vi "试验判定.vi"(7 "Result":refnum<vi>, 10 "判定参数":T1, 11 "XY曲线":cluster{"X":dbl[], "Y":dbl[]}[](array[cluster])) -> (2 "判定项长度":i32, 3 "OK？":bool)   [LabVIEW 2020]
uses:
  Global_Variable/A131258.vi
  <userlib>/_MGI/1D Array/MGI Average/MGI Average (DBL[]).vi
panel:
  out "逆向平均值":dbl
  out "正向平均值":dbl
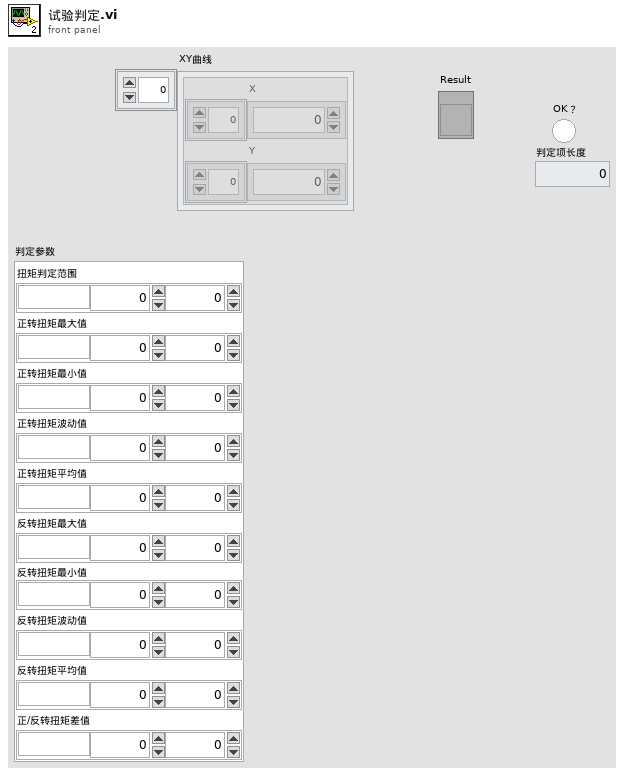
[diagram p1: front panel]
types:
  T1 = cluster{"扭矩判定范围":cluster{"单位":string, "下限":dbl, "上限":dbl}, "正转扭矩最大值":cluster{"单位":string, "下限":dbl, "上限":dbl}, "正转扭矩最小值":cluster{"单位":string, "下限":dbl, "上限":dbl}, "正转扭矩波动值":cluster{"单位":string, "下限":dbl, "上限":dbl}, "正转扭矩平均值":cluster{"单位":string, "下限":dbl, "上限":dbl}, "反转扭矩最大值":cluster{"单位":string, "下限":dbl, "上限":dbl}, "反转扭矩最小值":cluster{"单位":string, "下限":dbl, "上限":dbl}, "反转扭矩波动值":cluster{"单位":string, "下限":dbl, "上限":dbl}, "反转扭矩平均值":cluster{"单位":string, "下限":dbl, "上限":dbl}, "正/反转扭矩差值":cluster{"单位":string, "下限":dbl, "上限":dbl}}
  T2 = cluster{"左平均扭矩":cluster{"正转":dbl, "反转":dbl}, "左矩波动":cluster{"正转":dbl, "反转":dbl}, "左空载":cluster{"正转":dbl, "反转":dbl}, "右平均扭矩":cluster{"正转":dbl, "反转":dbl}, "右扭矩波动":cluster{"正转":dbl, "反转":dbl}, "右空载":cluster{"正转":dbl, "反转":dbl}, "扭矩对称":cluster{"左":dbl, "右":dbl}, "左零点漂移":cluster{"正":dbl, "反":dbl}, "右零点漂移":cluster{"正":dbl, "反":dbl}}
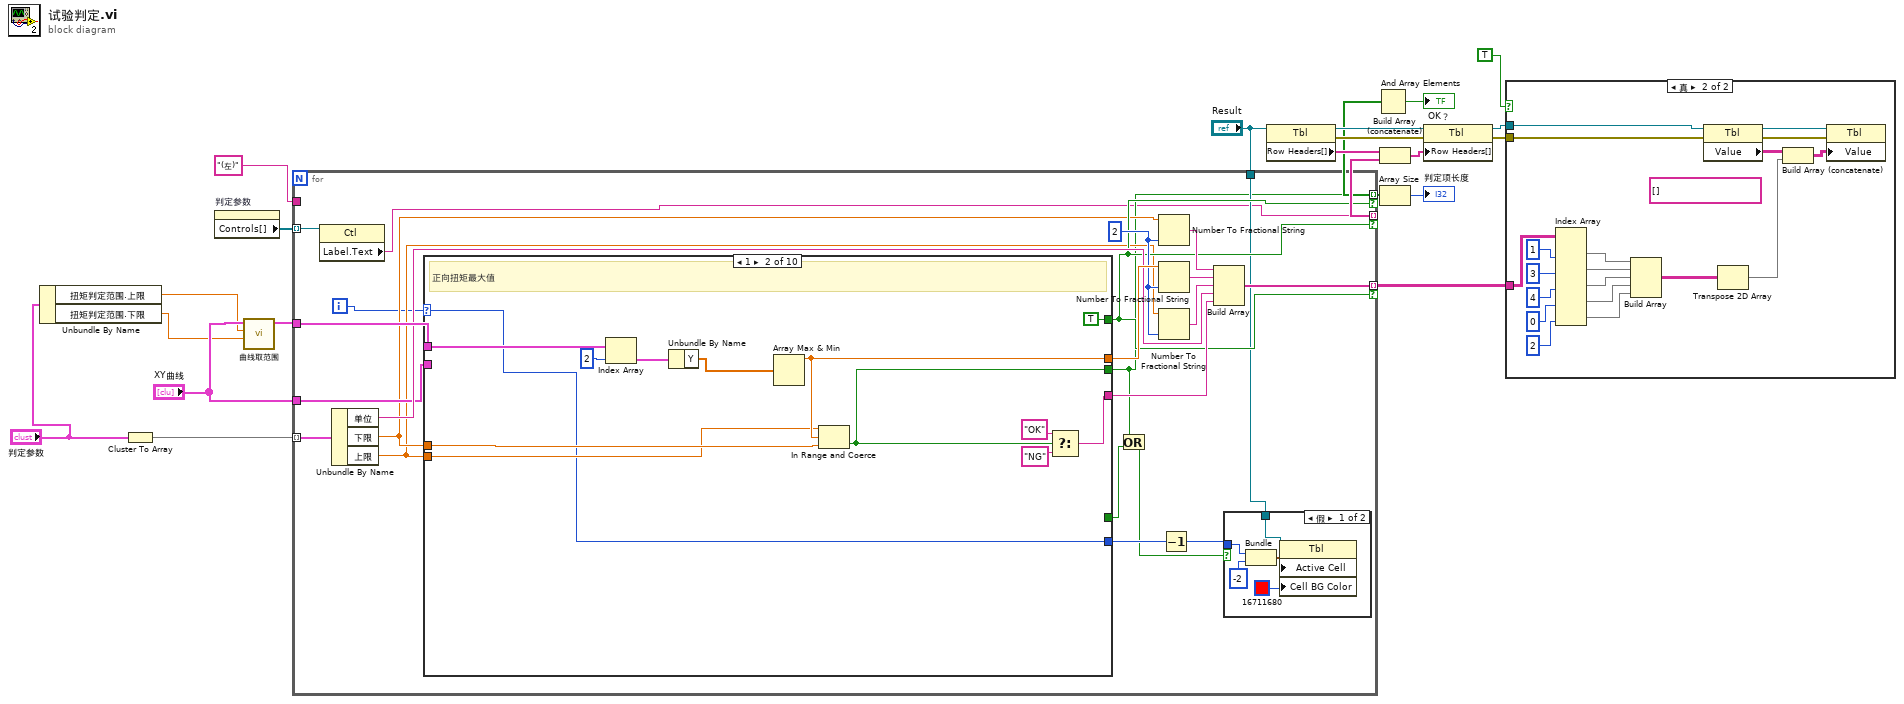
[diagram p0: block diagram]
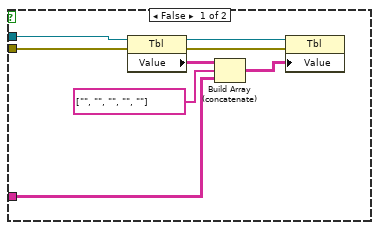
[diagram p2: hidden frame]
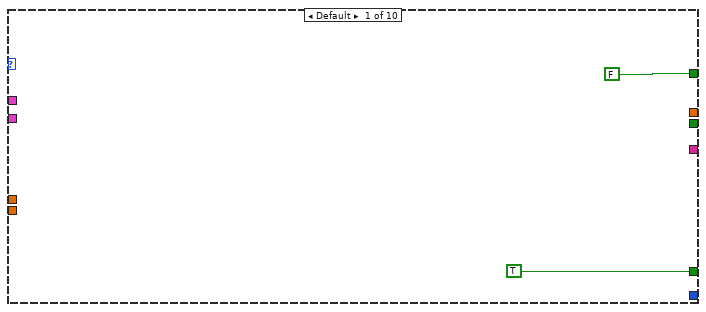
[diagram p4: hidden frame]
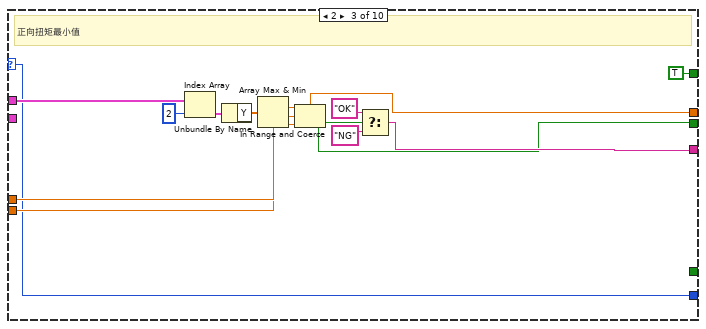
[diagram p5: hidden frame]
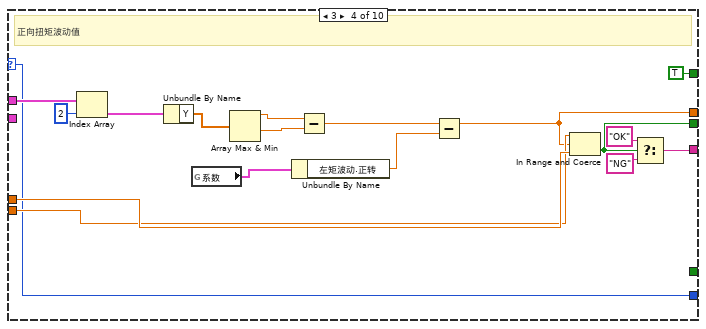
[diagram p6: hidden frame]
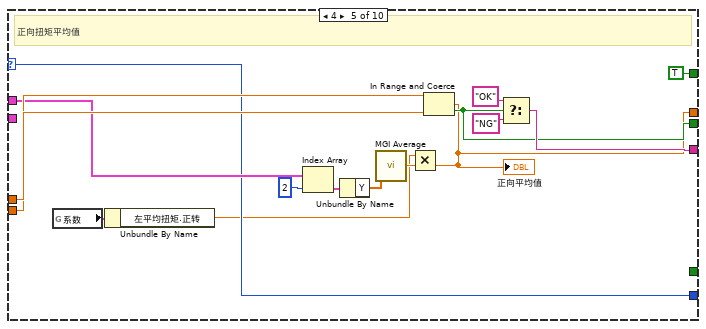
[diagram p7: hidden frame]
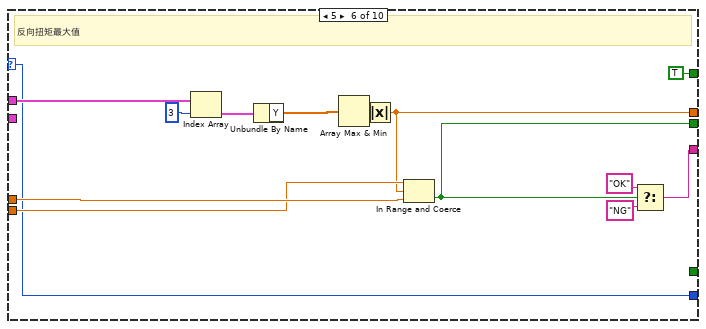
[diagram p8: hidden frame]
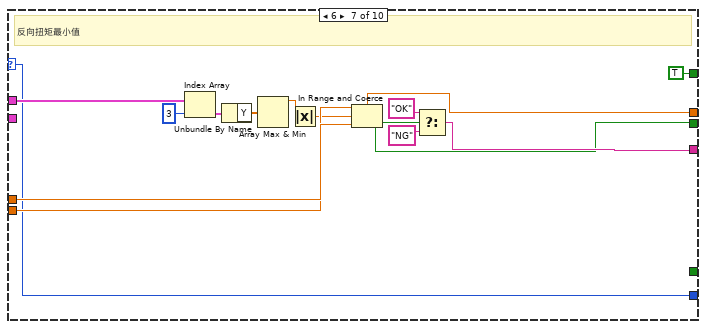
[diagram p9: hidden frame]
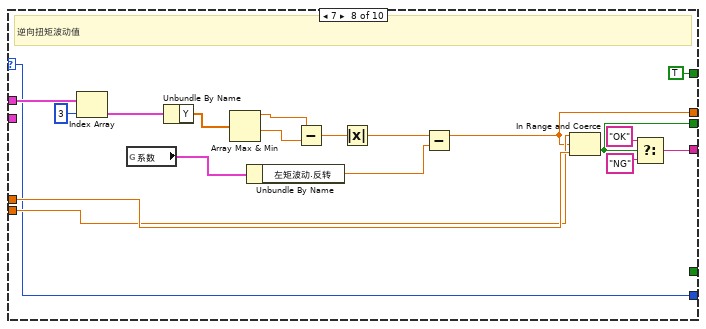
[diagram p10: hidden frame]
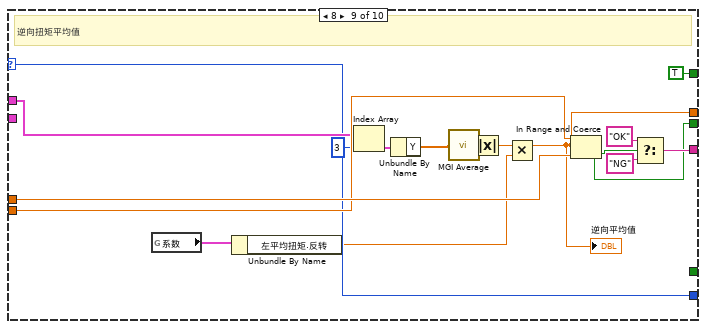
[diagram p11: hidden frame]
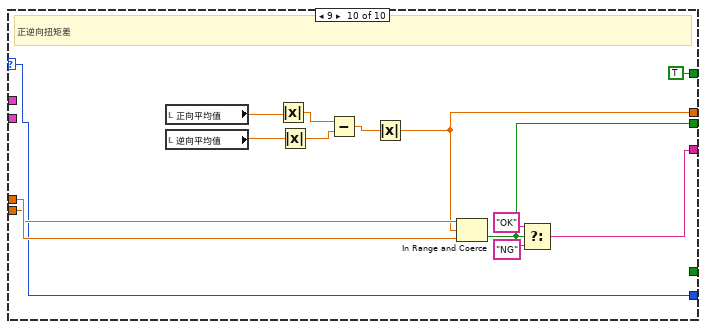
[diagram p12: hidden frame]
diagram:
  n1 = Unbundle By Name("判定参数") -> ("扭矩判定范围.上限"=w2:dbl, "扭矩判定范围.下限"=w3:dbl)
  n2 = Cluster To Array(cluster="判定参数") -> (array=w21:cluster{"单位":string, "下限":dbl, "上限":dbl}[])
  n3 = property on="判定参数" class="Clust (严格)"() -> ("Controls[]"=w11:refnum<vi>[])  [unwired: 2 in, 2 out]
  n4 = call "曲线取范围.vi"("下限"=w3, "上限"=w2, "曲线In"="XY曲线") -> ("曲线Out"=w5:cluster{"X":dbl[], "Y":dbl[]}[])  [unwired: 8 in]
  n5 = for {
    tunnel: w21 -> [w44] mode=indexing
    tunnel: w11 -> [w43] mode=indexing
    tunnel: w5 -> [w41]
    tunnel: [w28] -> w9 mode=indexing if=w33
    tunnel: [w34] -> w12 mode=indexing if=w33
    tunnel: [w24] -> w14 mode=indexing if=w33
    tunnel: "XY曲线" -> [w32]
    tunnel: "(左)" ("Label.Text") -> [_]
    tunnel: "Result" -> [w29]
    i -> [w23]
    w40 = i16 2 ("精度(6)")
    n6 = property class="Ctl"(reference=w43) -> ("Label.Text"=w24:string)  [unwired: 1 in, 2 out]
    n7 = Unbundle By Name(w44) -> ("单位"=w35:string, "下限"=w31:dbl, "上限"=w30:dbl)
    n8 = case shown="1" w23 {
      selector: w23 -> [_ w53 w66 w82 w100 w115 w129 w145 w164 w177]
      tunnel: [_ w61 w69 w79 w97 w113 w127 w141 w160 w178] -> w42
      tunnel: w41 -> [_ w64 w77 w89 w105 w125 w139 w152 w169 _]
      tunnel: [_ w58 w73 w93 w109 w120 w135 w156 w173 w179] -> w36
      tunnel: [_ w52 w65 w81 w99 w112 w126 w143 w162 w176] -> w28
      tunnel: w31 -> [_ w57 w72 w92 w108 w119 w134 w155 w172 w186]
      tunnel: w30 -> [_ w56 w71 w91 w107 w118 w133 w154 w171 w185]
      tunnel: [FALSE TRUE TRUE TRUE TRUE TRUE TRUE TRUE TRUE TRUE] -> w33
      tunnel: w32 -> [_ _ _ _ _ _ _ _ _ _]
      tunnel: [_ w53 w66 w82 w100 w115 w129 w145 w164 w177] -> w27
      tunnel: [TRUE _ _ _ _ _ _ _ _ _] -> w25
      frame Default {
      }
      frame 1 {
        # "正向扭矩最大值"
        n9 = Index Array(array=w64, index=2 ("索引")) -> (element=w62:cluster{"X":dbl[], "Y":dbl[]})
        n10 = Unbundle By Name(w62) -> ("Y"=w54:dbl[])
        n11 = Array Max & Min(array=w54) -> (max value=w61:dbl)  [unwired: 3 out]
        n12 = In Range and Coerce(upper limit=w56, x=w61, lower limit=w57) -> (In Range?=w52:bool)  [unwired: 1 out]
        n13 = Select(t="OK", s=w52, f="NG") -> (s? t:f=w58:string)
      }
      frame 2 {
        # "正向扭矩最小值"
        n14 = Index Array(array=w77, index=2 ("索引")) -> (element=w76:cluster{"X":dbl[], "Y":dbl[]})
        n15 = Unbundle By Name(w76) -> ("Y"=w68:dbl[])
        n16 = Array Max & Min(array=w68) -> (min value=w69:dbl)  [unwired: 3 out]
        n17 = In Range and Coerce(upper limit=w71, x=w69, lower limit=w72) -> (In Range?=w65:bool)  [unwired: 1 out]
        n18 = Select(t="OK", s=w65, f="NG") -> (s? t:f=w73:string)
      }
      frame 3 {
        # "正向扭矩波动值"
        n19 = Index Array(array=w89, index=2 ("索引")) -> (element=w88:cluster{"X":dbl[], "Y":dbl[]})
        n20 = Unbundle By Name(w88) -> ("Y"=w86:dbl[])
        n21 = global read "A131258.vi" "系数"() -> (w80:T2)
        n22 = Array Max & Min(array=w86) -> (max value=w85:dbl, min value=w84:dbl)  [unwired: 2 out]
        n23 = Unbundle By Name(w80) -> ("左矩波动.正转"=w78:dbl)
        n24 = Subtract(x=w85, y=w84) -> (x-y=w83:dbl)
        n25 = Subtract(x=w83, y=w78) -> (x-y=w79:dbl)
        n26 = In Range and Coerce(upper limit=w91, x=w79, lower limit=w92) -> (In Range?=w81:bool)  [unwired: 1 out]
        n27 = Select(t="OK", s=w81, f="NG") -> (s? t:f=w93:string)
      }
      frame 4 {
        # "正向扭矩平均值"
        n28 = global read "A131258.vi" "系数"() -> (w98:T2)
        n29 = Unbundle By Name(w98) -> ("左平均扭矩.正转"=w96:dbl)
        n30 = Index Array(array=w105, index=2 ("索引")) -> (element=w104:cluster{"X":dbl[], "Y":dbl[]})
        n31 = Unbundle By Name(w104) -> ("Y"=w101:dbl[])
        n32 = call-poly <userlib>:"MGI Average.vi"("Double[]"=w101) -> ("Average"=w102:dbl)  [unwired: 1 in]
        n33 = Multiply(x=w96, y=w102) -> (x*y=w97:dbl)
        "正向平均值" <- w97
        n34 = In Range and Coerce(upper limit=w107, x=w97, lower limit=w108) -> (In Range?=w99:bool)  [unwired: 1 out]
        n35 = Select(t="OK", s=w99, f="NG") -> (s? t:f=w109:string)
      }
      frame 5 {
        # "反向扭矩最大值"
        n36 = Index Array(array=w125, index=3 ("索引")) -> (element=w123:cluster{"X":dbl[], "Y":dbl[]})
        n37 = Unbundle By Name(w123) -> ("Y"=w116:dbl[])
        n38 = Array Max & Min(array=w116) -> (min value=w114:dbl)  [unwired: 3 out]
        n39 = Absolute Value(x=w114) -> (abs(x)=w113:dbl)
        n40 = In Range and Coerce(upper limit=w118, x=w113, lower limit=w119) -> (In Range?=w112:bool)  [unwired: 1 out]
        n41 = Select(t="OK", s=w112, f="NG") -> (s? t:f=w120:string)
      }
      frame 6 {
        # "反向扭矩最小值"
        n42 = Index Array(array=w139, index=3 ("索引")) -> (element=w138:cluster{"X":dbl[], "Y":dbl[]})
        n43 = Unbundle By Name(w138) -> ("Y"=w131:dbl[])
        n44 = Array Max & Min(array=w131) -> (max value=w128:dbl)  [unwired: 3 out]
        n45 = Absolute Value(x=w128) -> (abs(x)=w127:dbl)
        n46 = In Range and Coerce(upper limit=w133, x=w127, lower limit=w134) -> (In Range?=w126:bool)  [unwired: 1 out]
        n47 = Select(t="OK", s=w126, f="NG") -> (s? t:f=w135:string)
      }
      frame 7 {
        # "逆向扭矩波动值"
        n48 = Index Array(array=w152, index=3 ("索引")) -> (element=w151:cluster{"X":dbl[], "Y":dbl[]})
        n49 = global read "A131258.vi" "系数"() -> (w142:T2)
        n50 = Unbundle By Name(w151) -> ("Y"=w149:dbl[])
        n51 = Array Max & Min(array=w149) -> (max value=w148:dbl, min value=w147:dbl)  [unwired: 2 out]
        n52 = Unbundle By Name(w142) -> ("左矩波动.反转"=w140:dbl)
        n53 = Subtract(x=w148, y=w147) -> (x-y=w146:dbl)
        n54 = Absolute Value(x=w146) -> (abs(x)=w144:dbl)
        n55 = Subtract(x=w144, y=w140) -> (x-y=w141:dbl)
        n56 = In Range and Coerce(upper limit=w154, x=w141, lower limit=w155) -> (In Range?=w143:bool)  [unwired: 1 out]
        n57 = Select(t="OK", s=w143, f="NG") -> (s? t:f=w156:string)
      }
      frame 8 {
        # "逆向扭矩平均值"
        n58 = global read "A131258.vi" "系数"() -> (w161:T2)
        n59 = Unbundle By Name(w161) -> ("左平均扭矩.反转"=w159:dbl)
        n60 = Index Array(array=w169, index=3 ("索引")) -> (element=w168:cluster{"X":dbl[], "Y":dbl[]})
        n61 = Unbundle By Name(w168) -> ("Y"=w167:dbl[])
        n62 = call-poly <userlib>:"MGI Average.vi"("Double[]"=w167) -> ("Average"=w165:dbl)  [unwired: 1 in]
        n63 = Absolute Value(x=w165) -> (abs(x)=w163:dbl)
        n64 = Multiply(x=w163, y=w159) -> (x*y=w160:dbl)
        "逆向平均值" <- w160
        n65 = In Range and Coerce(upper limit=w171, x=w160, lower limit=w172) -> (In Range?=w162:bool)  [unwired: 1 out]
        n66 = Select(t="OK", s=w162, f="NG") -> (s? t:f=w173:string)
      }
      frame 9 {
        # "正逆向扭矩差"
        n67 = local read "正向平均值"() -> (w184:dbl)
        n68 = local read "逆向平均值"() -> (w183:dbl)
        n69 = Absolute Value(x=w184) -> (abs(x)=w182:dbl)
        n70 = Absolute Value(x=w183) -> (abs(x)=w181:dbl)
        n71 = Subtract(x=w182, y=w181) -> (x-y=w180:dbl)
        n72 = Absolute Value(x=w180) -> (abs(x)=w178:dbl)
        n73 = In Range and Coerce(upper limit=w185, x=w178, lower limit=w186) -> (In Range?=w176:bool)  [unwired: 1 out]
        n74 = Select(t="OK", s=w176, f="NG") -> (s? t:f=w179:string)
      }
    }
    n75 = Or(x=w28, y=w25) -> (x .or. y?=w26:bool)
    n76 = Number To Fractional String(number=w31, precision (6)=w40) -> (F-format string=w39:string)  [unwired: 2 in]
    n77 = Number To Fractional String(number=w42, precision (6)=w40) -> (F-format string=w38:string)  [unwired: 2 in]
    n78 = Number To Fractional String(number=w30, precision (6)=w40) -> (F-format string=w37:string)  [unwired: 2 in]
    n79 = Decrement(x=w27) -> (x-1=w22:i32)
    n80 = Build Array(w39, w38, w37, w35, w36) -> (w34:string[])
    n81 = case shown="假" w26 {
      tunnel: w29 -> [w49 _]
      tunnel: w22 -> [w45 _]
      frame False {
        n82 = Bundle(w45, -2) -> (w47:cluster{i32, i32})  [unwired: 1 in]
        n83 = property class="Tbl"(reference=w49, "Active Cell"=w47, "Cell BG Color"=u32 16711680 ("活动单元格:单元格背景色")) -> ()  [unwired: 1 in, 2 out]
      }
      frame True {
      }
    }
  }
  n84 = property class="Tbl"(reference="Result") -> (reference out=w16:refnum<vi>, error out=w19:errorcluster, "Row Headers[]"=w13:string[])  [unwired: 1 in]
  n85 = And Array Elements(Boolean array=w9) -> (logical AND=→"OK？":bool)
  n86 = Build Array (concatenate)(w13, w14) -> (w15:string[])
  n87 = Array Size(array=w9) -> (size(s)=→"判定项长度":i32)
  n88 = property class="Tbl"(reference=w16, error in=w19, "Row Headers[]"=w15) -> (reference out=w17:refnum<vi>, error out=w18:errorcluster)
  n89 = case shown="真" TRUE {
    tunnel: w18 -> [w195 w214]
    tunnel: w17 -> [w192 w211]
    tunnel: w12 -> [w191 w210]
    frame False {
      n90 = property class="Tbl"(reference=w192, error in=w195) -> (reference out=w193:refnum<vi>, error out=w194:errorcluster, "Value"=w196:string[][])
      n91 = Build Array (concatenate)(w196, string[] ["", "", "", "", ""], w191) -> (w197:string[][])
      n92 = property class="Tbl"(reference=w193, error in=w194, "Value"=w197) -> ()  [unwired: 2 out]
    }
    frame True {
      (unwired) string[] []
      n93 = Index Array(array=w210, index (col) #1=1 ("禁用的索引 (列)"), index (col) #2=3 ("索引 (列)"), index (col) #3=4 ("索引 (列)"), index (col) #4=0 ("索引 (列)"), index (col) #5=2 ("索引 (列)")) -> (element #1=w206:string[], element #2=w205:string[], element #3=w204:string[], element #4=w199:string[], element #5=w198:string[])  [unwired: 5 in]
      n94 = Build Array(w206, w205, w204, w199, w198) -> (w203:string[][])
      n95 = property class="Tbl"(reference=w211, error in=w214) -> (reference out=w212:refnum<vi>, error out=w213:errorcluster, "Value"=w215:string[][])
      n96 = Transpose 2D Array(2D array=w203) -> (transposed array=w202:string[][])
      n97 = Build Array (concatenate)(w215, w202) -> (w216:string[][])
      n98 = property class="Tbl"(reference=w212, error in=w213, "Value"=w216) -> ()  [unwired: 2 out]
    }
  }
